vi "REC_magnet move program.vi"(4 "exp fit":cluster{"A":dbl, "B":dbl}={"A"=28.47, "B"=-1.501}, 5 "暂停磁铁引用":refnum<vi>, 6 "单次反馈":bool, 7 "反馈引用":refnum<vi>, 8 "预估时间引用":refnum<vi>, 9 "mag ctl":T1 {"磁铁运动参数"."FR每步时间(s)" min=0.5; "磁铁运动参数"."加载率(pN/s)" min=0.01}, 10 "停止测量引用":refnum<vi>, 11 "磁铁位置引用":refnum<vi>) -> (3 "完成测量":bool)   [LabVIEW 2017]
doc: "本VI是测量时控制磁铁运动的核心VI。\n不同的实验测量模式主要的区别就在于磁铁的运动过程不一样，因而在不同的测量模式下磁铁的运动模式也不同。\n必要的输入有：磁铁控制参数，临时终止测量，汇报磁铁位置。\n参数输入后首先会确定测量模式，然后敲定其他参数。\n目前完成的模式只有force clamp。\nFC的状态机逻辑如下：\n开始测量后，首先驰豫（可以设定驰豫位置），然后按位置数组和停留时间，顺序地走一遍，之后判断是否做往返，不做往返的话直接跳到完成检查阶段。如果做往返，跳转到返回运动，将数组反转后同样地走一遍，然后跳到完成检查阶段。完成检查阶段主要是判断是否测量了足够的周期，比如需要测两轮往返，那么在完成检查阶段就不会终止任务，而是跳转回到驰豫分支，开始一轮新的控制周期，直到完成了足够多的周期时，终止磁铁运动。"
uses:
  device control/magnet control.ctl
  device control/device index.ctl
  parameter set for record.ctl
  control/record mode.ctl
panel:
  # "force ramp"
  # "force ramp"
  # "通用"
  # "force ramp"
  # "force clamp"
  # "磁铁旋转"
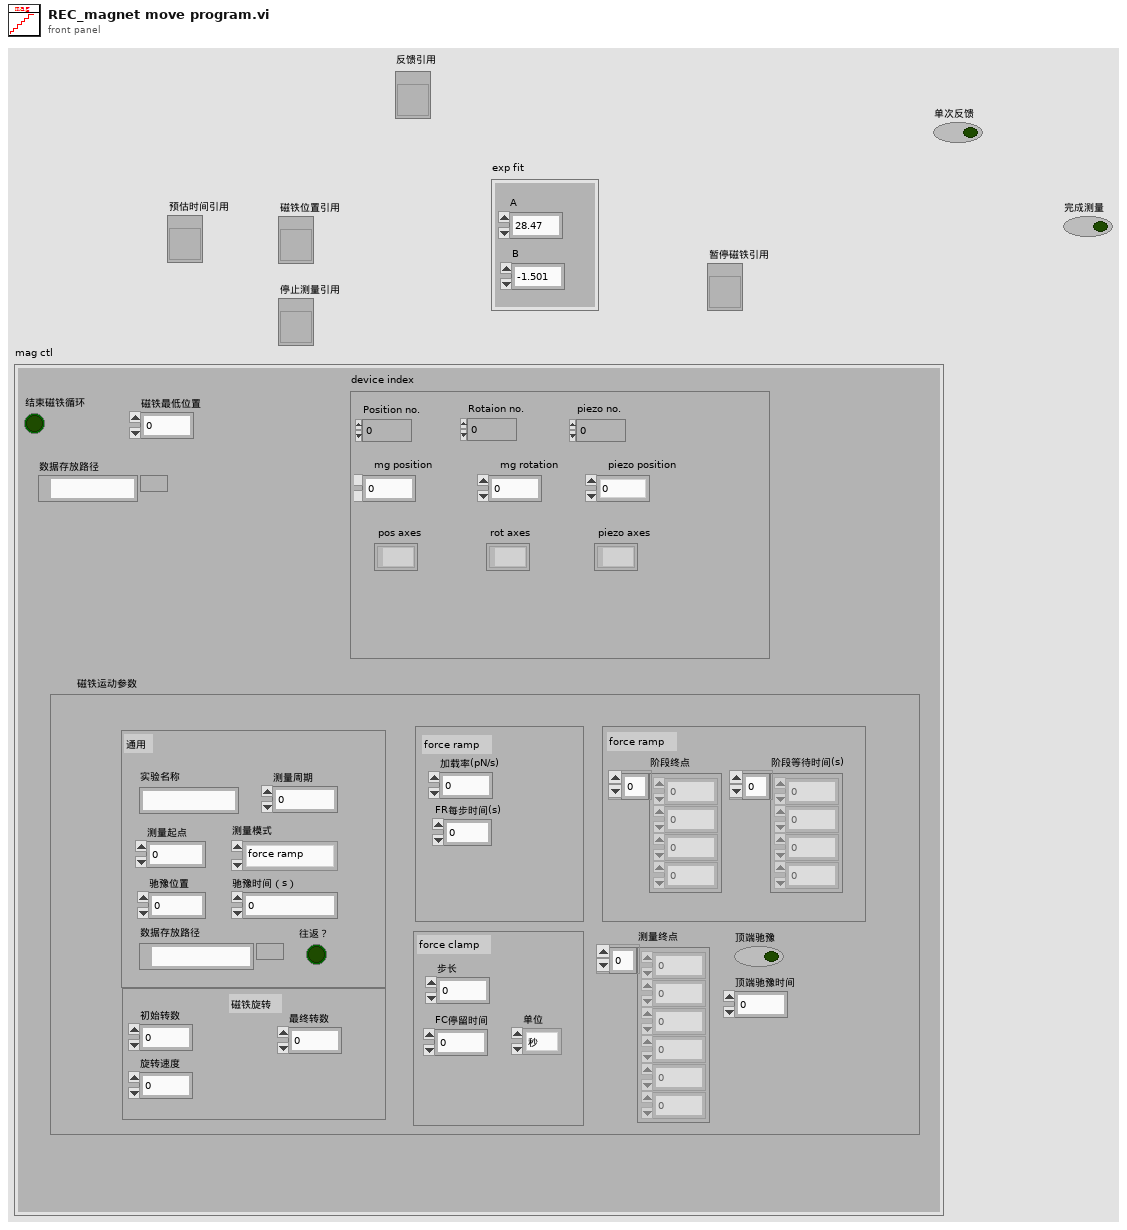
[diagram p1: front panel]
types:
  T1 = typedef "magnet control.ctl" = cluster{"device index":T2, "结束磁铁循环":bool, "磁铁最低位置":dbl, "数据存放路径":path, "磁铁运动参数":T3}
  T2 = typedef "device index.ctl" = cluster{"Position no.":i32, "Rotaion no.":i32, "piezo no.":i32, "mg position":dbl, "mg rotation":dbl, "piezo position":dbl, "pos axes":string[], "rot axes":string[], "piezo axes":string[]}
  T3 = typedef "parameter set for record.ctl" = cluster{"测量模式":T4, "测量起点":dbl, "数据存放路径":path, "加载率(pN/s)":dbl, "初始转数":dbl, "最终转数":dbl, "旋转速度":dbl, "步长":dbl, "FC停留时间":dbl, "实验名称":string, "往返？":bool, "驰豫时间（s）":dbl, "单位":enum16{"秒", "毫秒", "分"}, "测量周期":i32, "驰豫位置":dbl, "FR每步时间(s)":dbl, "测量终点":dbl[], "阶段终点":dbl[], "阶段等待时间(s)":dbl[], "顶端驰豫时间":u32, "顶端驰豫":bool}
  T4 = typedef "record mode.ctl" = enum16{"force ramp", "force clamp", "user-defined", "force-mixed"}
  T5 = typedef "磁铁进程控制变量.ctl" = enum16{"驰豫", "顺序运动", "返回运动", "完成检查"}
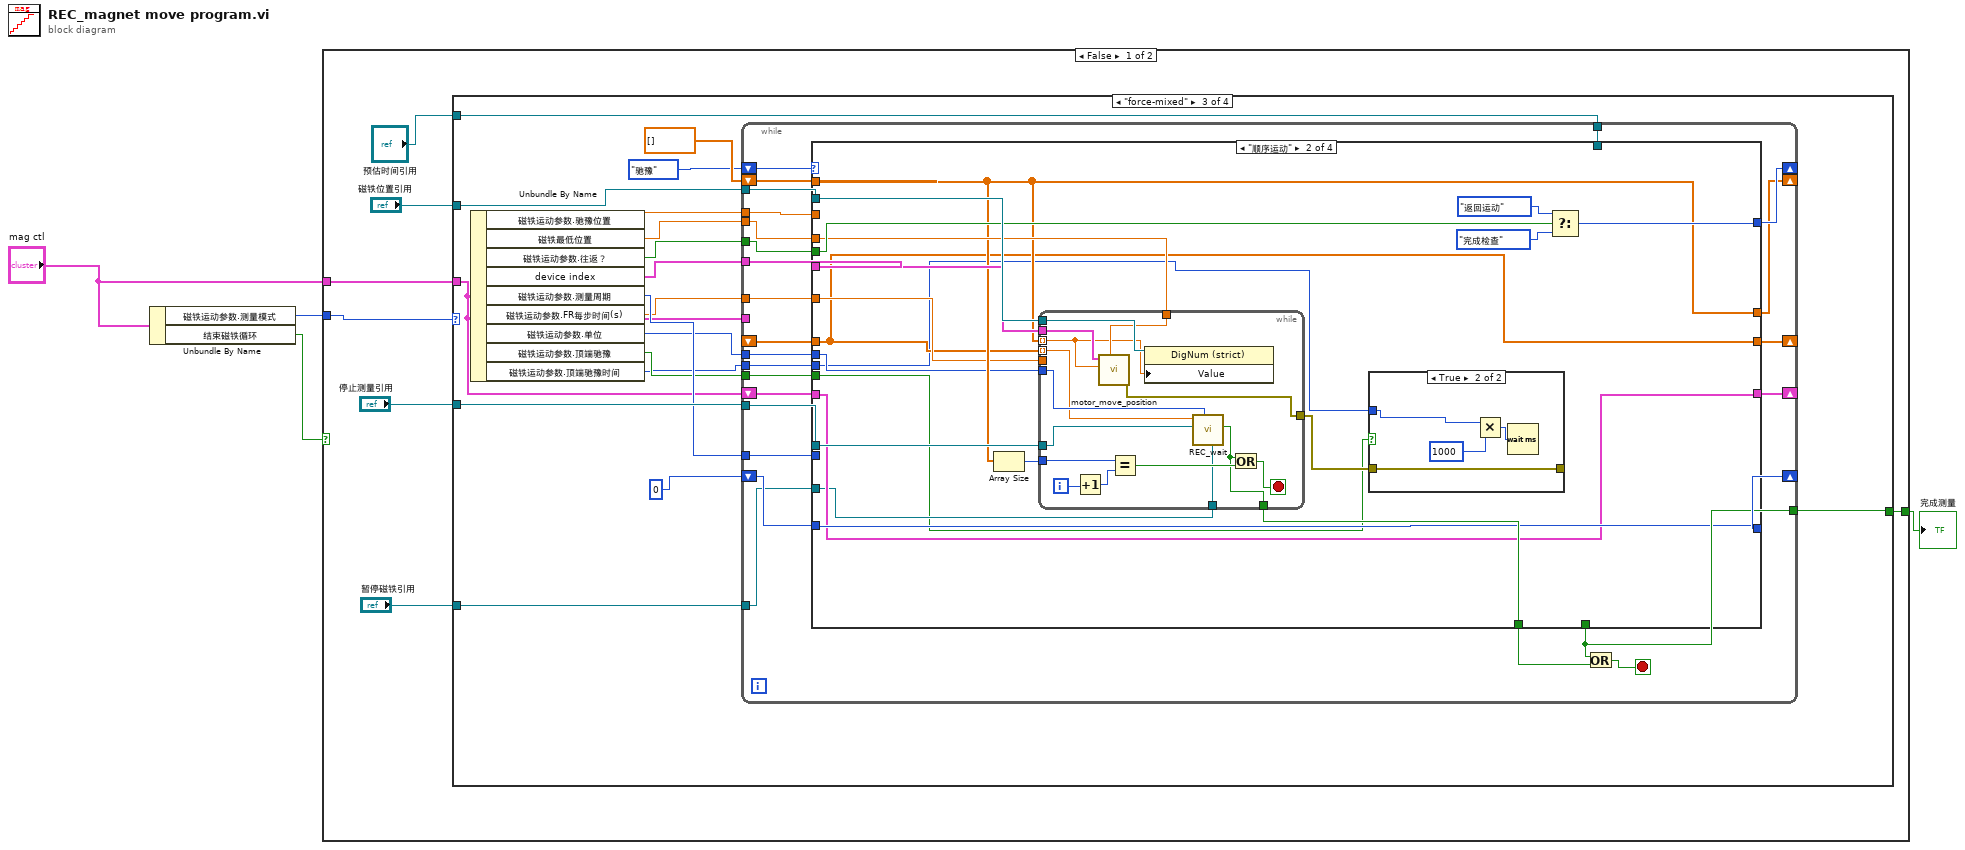
[diagram p0: block diagram]
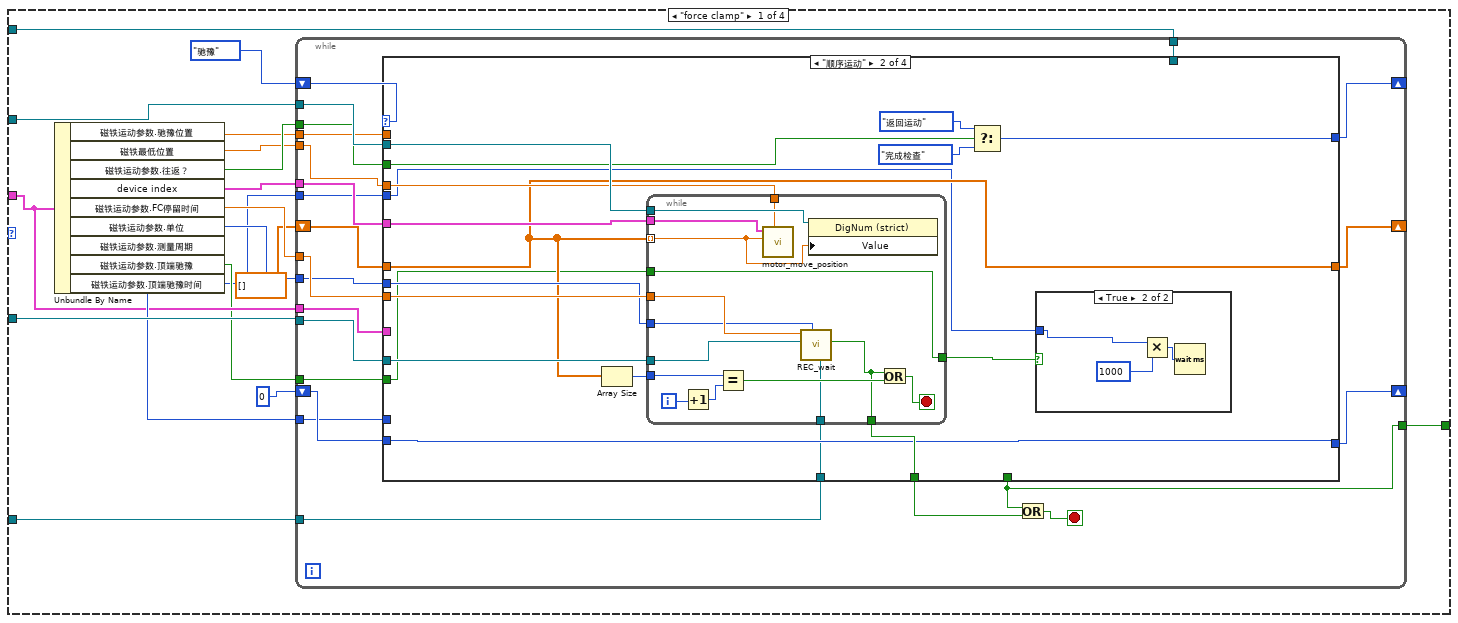
[diagram p2: hidden frame]
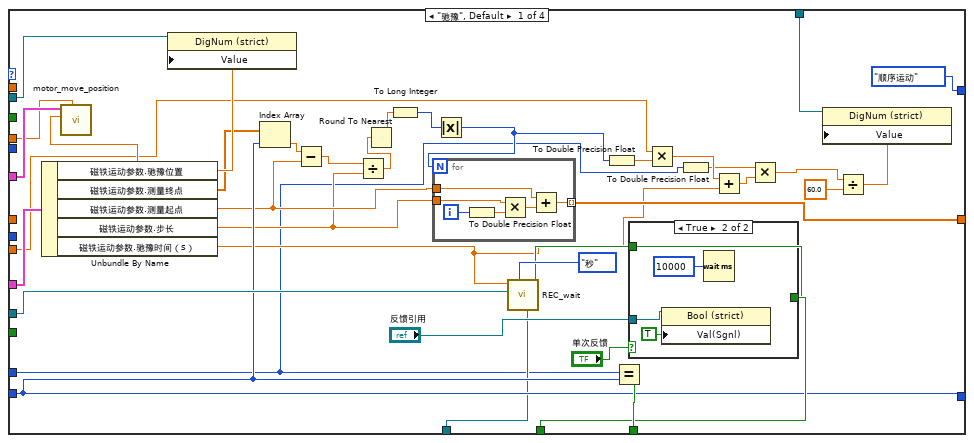
[diagram p3: hidden frame]
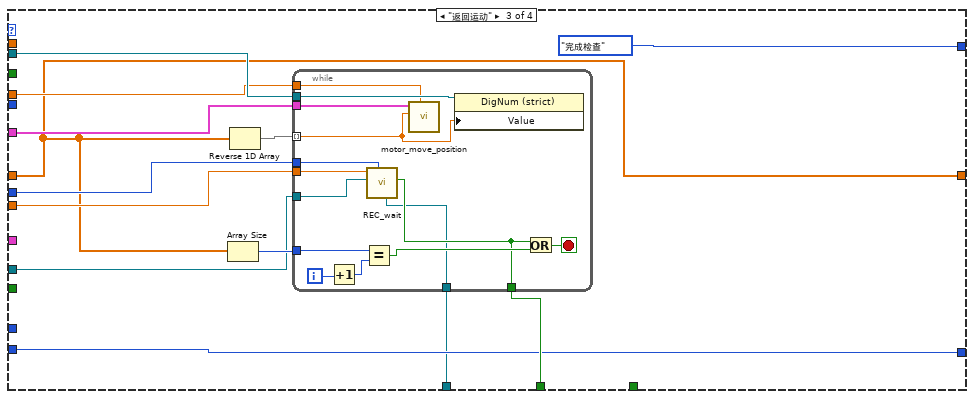
[diagram p6: hidden frame]
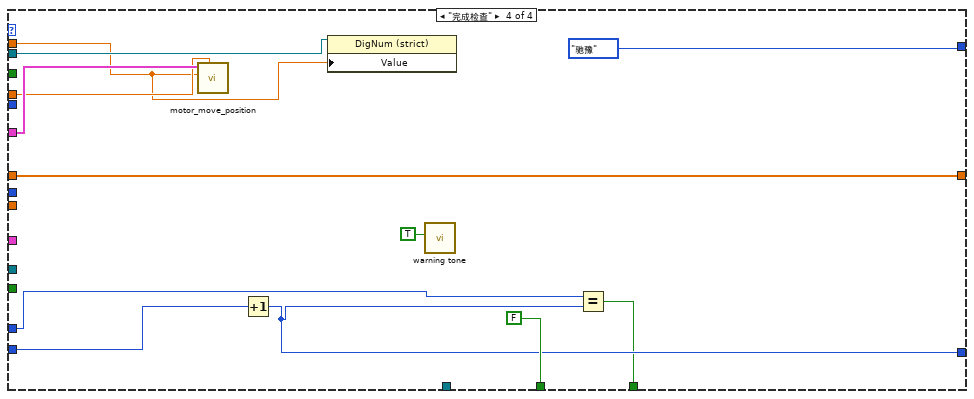
[diagram p7: hidden frame]
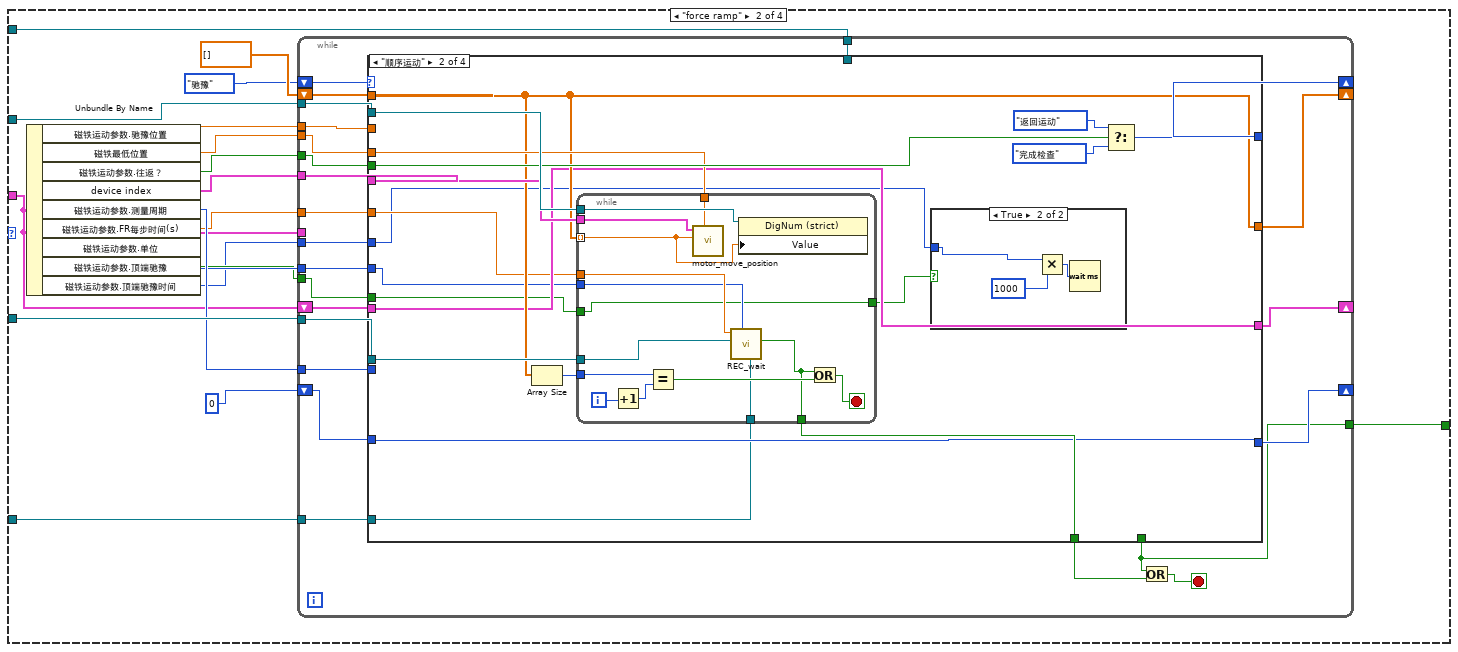
[diagram p8: hidden frame]
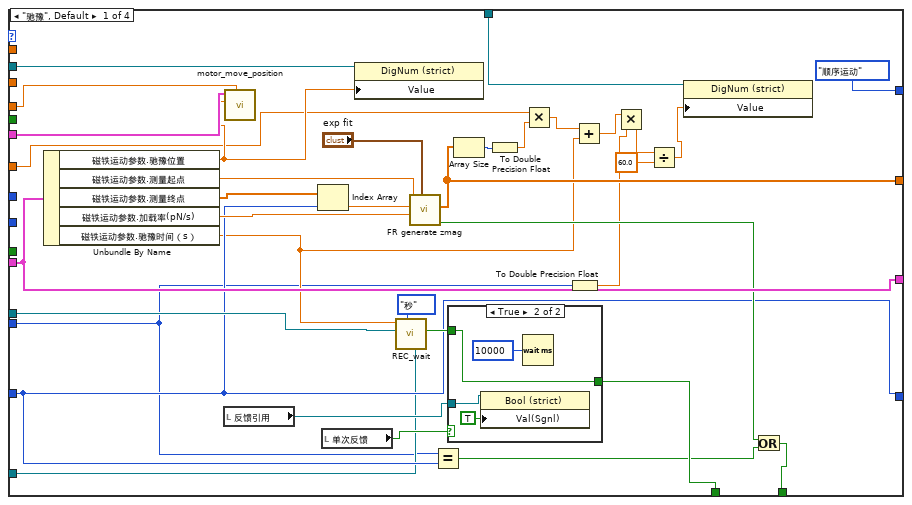
[diagram p9: hidden frame]
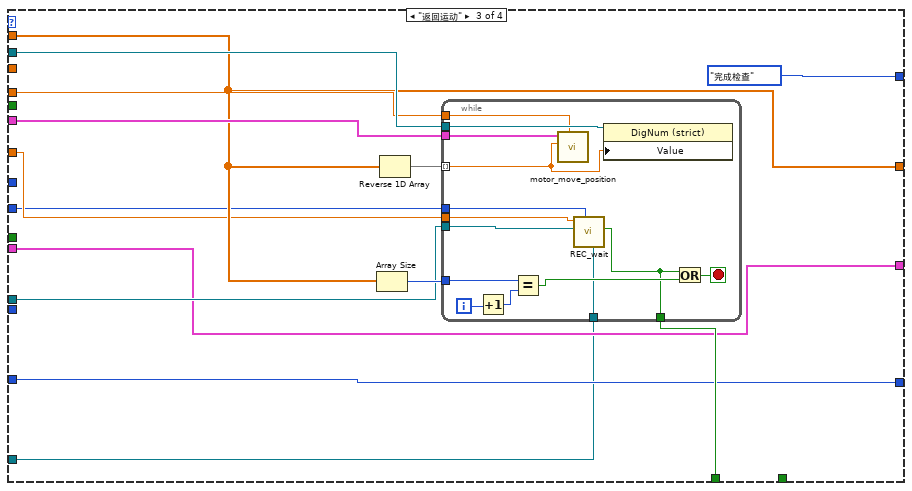
[diagram p12: hidden frame]
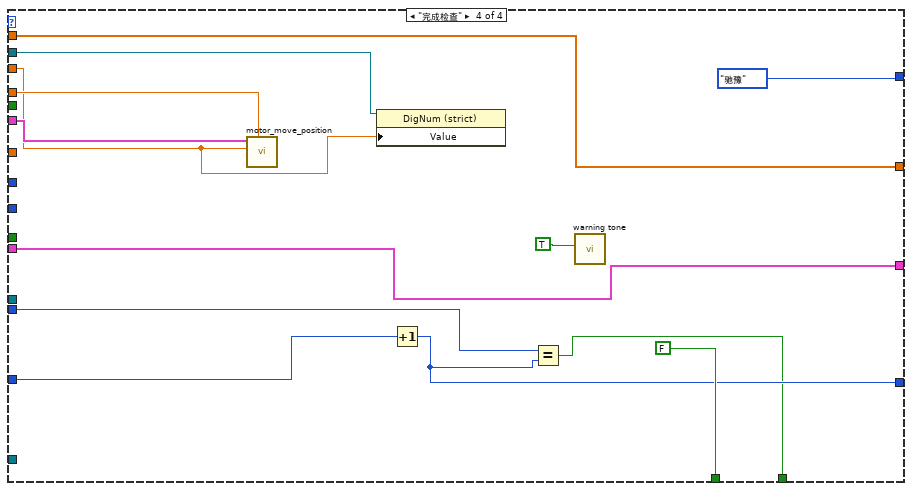
[diagram p13: hidden frame]
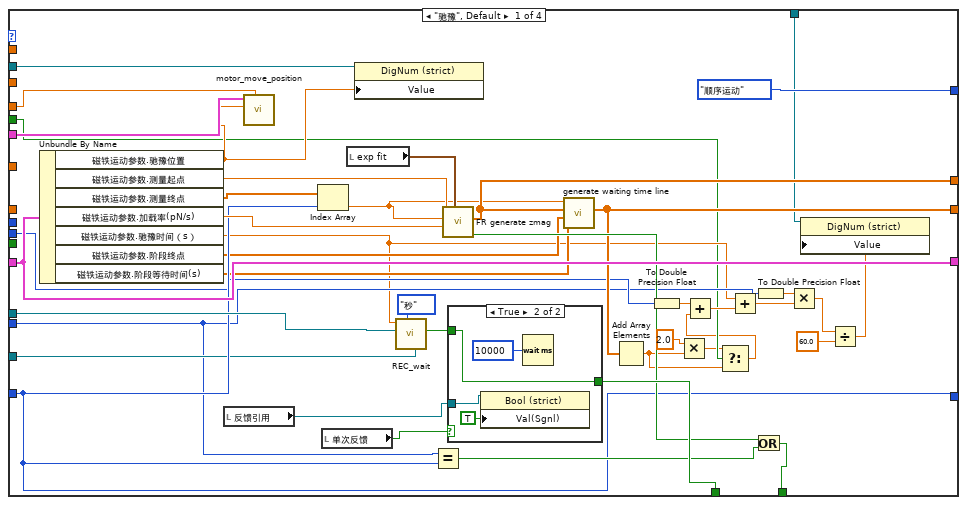
[diagram p14: hidden frame]
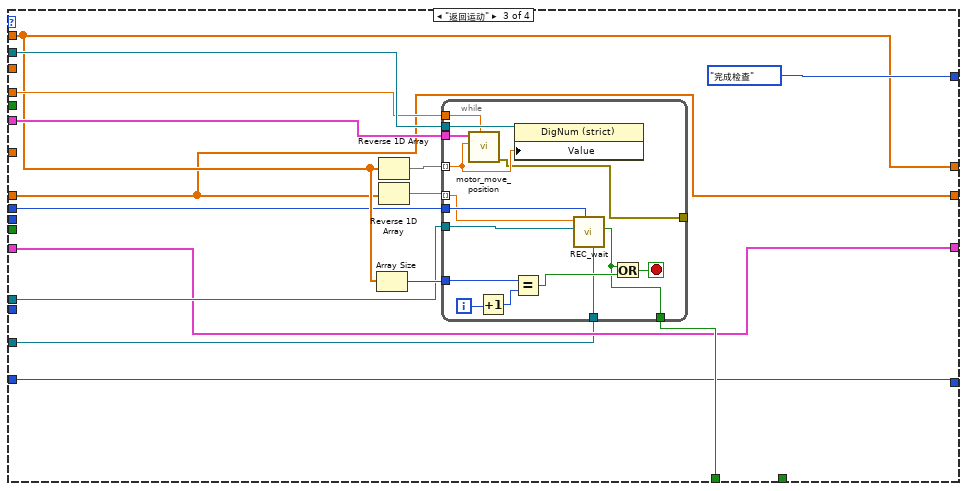
[diagram p17: hidden frame]
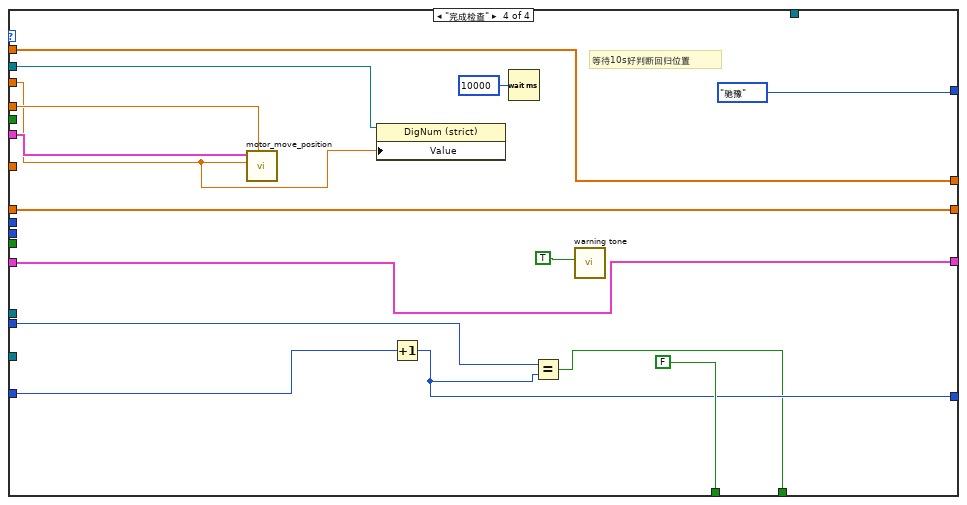
[diagram p18: hidden frame]
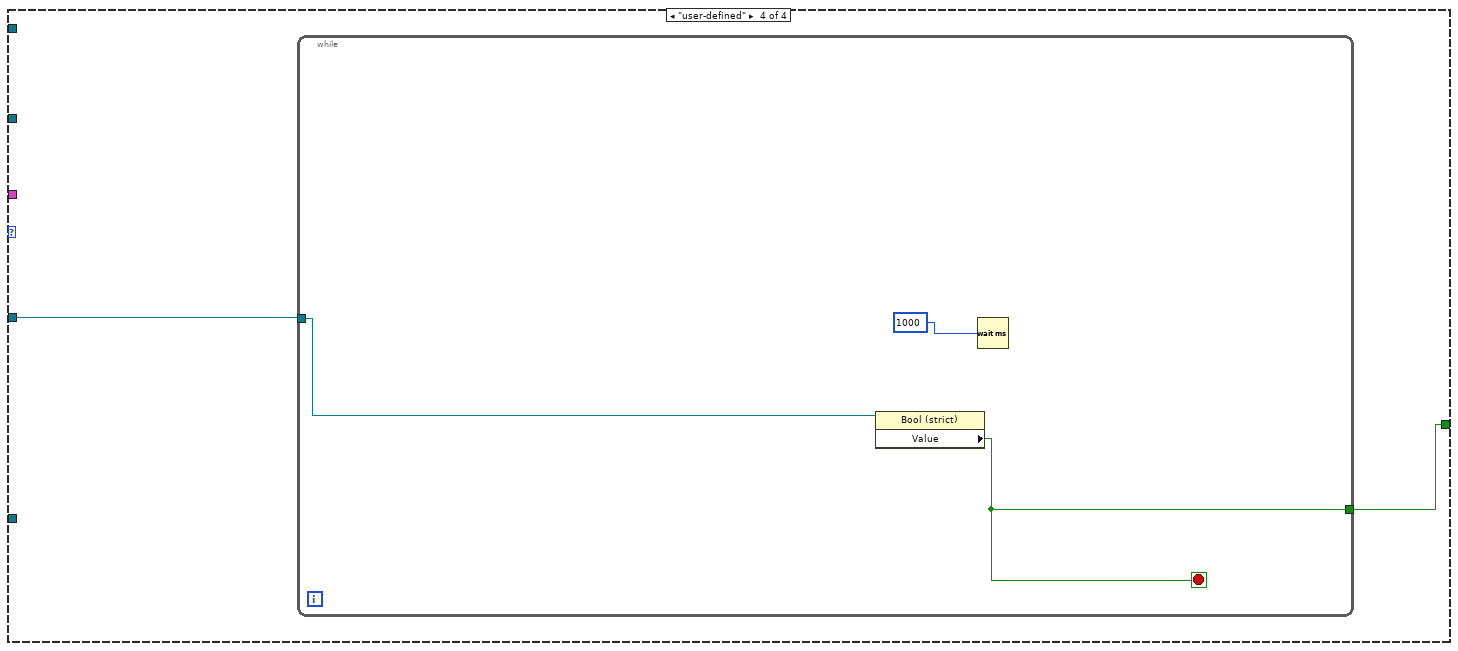
[diagram p19: hidden frame]
diagram:
  n1 = Unbundle By Name("mag ctl") -> ("磁铁运动参数.测量模式"=w4:T4, "结束磁铁循环"=w2:bool)
  n2 = case shown="False" w2 {
    selector: w2 -> [_ w516]
    tunnel: w4 -> [w11 _]
    tunnel: [w8 w516] -> w3
    tunnel: "mag ctl" -> [w7 _]
    frame False {
      n3 = case shown="\"force-mixed\"" w11 {
        tunnel: "磁铁位置引用" -> [w29 w189 w349 _]
        tunnel: "停止测量引用" -> [w28 w188 w348 w512]
        tunnel: w7 -> [w16 w183 w343 _]
        tunnel: [w21 w180 w340 w511] -> w8
        tunnel: "暂停磁铁引用" -> [w15 w178 w338 _]
        tunnel: "预估时间引用" -> [w14 w177 w335 _]
        frame "force clamp" {
          n4 = Unbundle By Name(w16) -> ("磁铁运动参数.驰豫位置"=w17:dbl, "磁铁最低位置"=w22:dbl, "磁铁运动参数.往返？"=w24:bool, "device index"=w26:T2, "磁铁运动参数.FC停留时间"=w25:dbl, "磁铁运动参数.单位"=w20:enum16{"秒", "毫秒", "分"}, "磁铁运动参数.测量周期"=w18:i32, "磁铁运动参数.顶端驰豫"=w13:bool, "磁铁运动参数.顶端驰豫时间"=w12:u32)
          n5 = while {
            tunnel: w29 -> [w52]
            tunnel: w28 -> [w51]
            shift-right: [w48] -> _
            shift-left: 磁铁进程控制变量."驰豫" -> [w49]
            tunnel: w26 -> [w47]
            tunnel: w25 -> [w46]
            tunnel: w24 -> [w45]
            shift-right: [w43] -> _
            shift-left: 0 -> [w44]
            tunnel: w22 -> [w42]
            tunnel: [w41] -> w21
            tunnel: w20 -> [w40]
            shift-right: [w39] -> _
            shift-left: dbl[] [] -> [w38]
            tunnel: w18 -> [w36]
            tunnel: w17 -> [w35]
            tunnel: w16 -> [w34]
            tunnel: w15 -> [w33]
            tunnel: w14 -> [w32]
            tunnel: w13 -> [w31]
            tunnel: w12 -> [w30]
            stop <- w50 stop-if-true
            n6 = case shown="\"顺序运动\"" w49 {
              tunnel: w52 -> [w84 w116 w142 w165]
              tunnel: w51 -> [w86 w115 w143 _]
              tunnel: [磁铁进程控制变量."顺序运动" w112 磁铁进程控制变量."完成检查" 磁铁进程控制变量."驰豫"] -> w48
              tunnel: [w81 w111 w146 FALSE ("Value")] -> w37
              tunnel: w47 -> [w85 w110 w144 w166]
              tunnel: w46 -> [w63 w109 w145 _]
              tunnel: w45 -> [_ w108 _ _]
              tunnel: w44 -> [w74 w107 w140 w172]
              tunnel: [w74 w107 w140 w169] -> w43
              tunnel: w42 -> [w83 w106 w139 w164]
              tunnel: [w82 _ _ w167] -> w41
              tunnel: w40 -> [_ w105 w138 _]
              tunnel: w34 -> [w68 _ _ _]
              tunnel: [w77 w104 w137 w171] -> w39
              tunnel: w38 -> [_ w104 w137 w171]
              tunnel: w36 -> [w58 _ _ w168]
              tunnel: w35 -> [_ _ _ w163]
              tunnel: w33 -> [w65 w103 w136 _]
              tunnel: w32 -> [w56 _ _ _]
              tunnel: w31 -> [_ w101 _ _]
              tunnel: w30 -> [_ w102 _ _]
              frame "驰豫", Default {
                n7 = Unbundle By Name(w68) -> ("磁铁运动参数.驰豫位置"=w78:dbl, "磁铁运动参数.测量终点"=w75:dbl[], "磁铁运动参数.测量起点"=w72:dbl, "磁铁运动参数.步长"=w71:dbl, "磁铁运动参数.驰豫时间（s）"=w64:dbl)
                n8 = call "motor_move_position.vi"("磁铁最低位置"=w83, "target position"=w78, "device index"=w85) -> ()  [unwired: 6 in, 3 out]
                n9 = property class="DigNum (strict)"(reference=w84, "Value"=w78) -> ()  [unwired: 1 in, 2 out]
                n10 = Index Array(array=w75, index=w74) -> (element=w73:dbl)
                n11 = Subtract(x=w73, y=w72) -> (x-y=w66:dbl)
                n12 = Divide(x=w66, y=w71) -> (x/y=w70:dbl)
                n13 = Round To Nearest(number=w70) -> (nearest integer value=w69:dbl)
                n14 = To Long Integer(number=w69) -> (32bit integer=w67:i32)
                n15 = Absolute Value(x=w67) -> (abs(x)=w62:i32)
                n16 = for {
                  N: w62 -> [_]
                  tunnel: w72 -> [w94]
                  tunnel: [w90] -> w77 mode=indexing
                  tunnel: w71 -> [w89]
                  i -> [w93]
                  n17 = To Double Precision Float(number=w93) -> (double precision float=w92:dbl)
                  n18 = Multiply(x=w89, y=w92) -> (x*y=w91:dbl)
                  n19 = Add(x=w94, y=w91) -> (x+y=w90:dbl)
                }
                n20 = call "REC_wait.vi"("暂停磁铁引用"=w65, "时间单位"=enum16{"秒", "毫秒", "分"}."秒", "停止测量引用"=w86, "停留时间"=w64) -> ("停止？"=w80:bool)  [unwired: 7 in]
                n21 = To Double Precision Float(number=w62) -> (double precision float=w61:dbl)
                n22 = Equal?(x=w58, y=w74) -> (x = y?=w82:bool)
                n23 = case shown="True" "单次反馈" {
                  selector: "单次反馈" -> [w95 _]
                  tunnel: [w95 w97] -> w81
                  tunnel: w80 -> [_ w97]
                  tunnel: "反馈引用" -> [_ w96]
                  frame False {
                  }
                  frame True {
                    n24 = property class="Bool (strict)"(reference=w96, "Val(Sgnl)"=TRUE ("值(信号)")) -> ()  [unwired: 1 in, 2 out]
                    n25 = Wait (ms)(milliseconds to wait=u32 10000 ("等待时间（毫秒）")) -> ()  [unwired: 1 out]
                  }
                }
                n26 = Multiply(x=w63, y=w61) -> (x*y=w60:dbl)
                n27 = To Double Precision Float(number=w58) -> (double precision float=w57:dbl)
                n28 = Add(x=w60, y=w64) -> (x+y=w59:dbl)
                n29 = Multiply(x=w57, y=w59) -> (x*y=w54:dbl)
                n30 = Divide(x=w54, y=60.0) -> (x/y=w53:dbl)
                n31 = property class="DigNum (strict)"(reference=w56, "Value"=w53) -> ()  [unwired: 1 in, 2 out]
              }
              frame "顺序运动" {
                n32 = Array Size(array=w104) -> (size(s)=w117:i32)
                n33 = while {
                  tunnel: w117 -> [w135]
                  tunnel: w116 -> [w130]
                  tunnel: w115 -> [w127]
                  tunnel: [w126] -> w111
                  tunnel: w110 -> [w129]
                  tunnel: w109 -> [w128]
                  tunnel: w106 -> [w125]
                  tunnel: w105 -> [w124]
                  tunnel: w104 -> [w123] mode=indexing
                  tunnel: w103 -> [w122]
                  tunnel: [w121] -> w100
                  tunnel: w101 -> [w121]
                  i -> [w134]
                  stop <- w132 stop-if-true
                  n34 = Increment(x=w134) -> (x+1=w133:i32)
                  n35 = Equal?(x=w135, y=w133) -> (x = y?=w131:bool)
                  n36 = call "motor_move_position.vi"("磁铁最低位置"=w125, "target position"=w123, "device index"=w129) -> ()  [unwired: 6 in, 3 out]
                  n37 = call "REC_wait.vi"("暂停磁铁引用"=w122, "时间单位"=w124, "停止测量引用"=w127, "停留时间"=w128) -> ("停止？"=w126:bool)  [unwired: 7 in]
                  n38 = property class="DigNum (strict)"(reference=w130, "Value"=w123) -> ()  [unwired: 1 in, 2 out]
                  n39 = Or(x=w126, y=w131) -> (x .or. y?=w132:bool)
                }
                n40 = Select(t=磁铁进程控制变量."返回运动", s=w108, f=磁铁进程控制变量."完成检查") -> (s? t:f=w112:T5)
                n41 = case shown="True" w100 {
                  tunnel: w102 -> [_ w118]
                  frame False {
                  }
                  frame True {
                    n42 = Multiply(x=w118, y=u32 1000) -> (x*y=w119:u32)
                    n43 = Wait (ms)(milliseconds to wait=w119) -> ()  [unwired: 1 out]
                  }
                }
              }
              frame "返回运动" {
                n44 = Array Size(array=w137) -> (size(s)=w147:i32)
                n45 = Reverse 1D Array(array=w137) -> (reversed array=w148:dbl[])
                n46 = while {
                  tunnel: [w153] -> w146
                  tunnel: w148 -> [w151] mode=indexing
                  tunnel: w147 -> [w158]
                  tunnel: w145 -> [w157]
                  tunnel: w144 -> [w156]
                  tunnel: w143 -> [w154]
                  tunnel: w142 -> [w155]
                  tunnel: w139 -> [w152]
                  tunnel: w138 -> [w150]
                  tunnel: w136 -> [w149]
                  i -> [w162]
                  stop <- w160 stop-if-true
                  n47 = Increment(x=w162) -> (x+1=w161:i32)
                  n48 = Equal?(x=w158, y=w161) -> (x = y?=w159:bool)
                  n49 = call "REC_wait.vi"("暂停磁铁引用"=w149, "时间单位"=w150, "停止测量引用"=w154, "停留时间"=w157) -> ("停止？"=w153:bool)  [unwired: 7 in]
                  n50 = call "motor_move_position.vi"("磁铁最低位置"=w152, "target position"=w151, "device index"=w156) -> ()  [unwired: 6 in, 3 out]
                  n51 = property class="DigNum (strict)"(reference=w155, "Value"=w151) -> ()  [unwired: 1 in, 2 out]
                  n52 = Or(x=w153, y=w159) -> (x .or. y?=w160:bool)
                }
              }
              frame "完成检查" {
                n53 = call "motor_move_position.vi"("磁铁最低位置"=w164, "target position"=w163, "device index"=w166) -> ()  [unwired: 6 in, 3 out]
                n54 = Increment(x=w172) -> (x+1=w169:i32)
                n55 = property class="DigNum (strict)"(reference=w165, "Value"=w163) -> ()  [unwired: 1 in, 2 out]
                n56 = call "warning tone.vi"("Ring?"=TRUE) -> ()  [unwired: 11 in]
                n57 = Equal?(x=w168, y=w169) -> (x = y?=w167:bool)
              }
            }
            n58 = Or(x=w41, y=w37) -> (x .or. y?=w50:bool)
          }
        }
        frame "force ramp" {
          n59 = Unbundle By Name(w183) -> ("磁铁运动参数.驰豫位置"=w179:dbl, "磁铁最低位置"=w191:dbl, "磁铁运动参数.往返？"=w190:bool, "device index"=w192:T2, "磁铁运动参数.测量周期"=w185:i32, "磁铁运动参数.FR每步时间(s)"=w182:dbl, "磁铁运动参数.单位"=w181:enum16{"秒", "毫秒", "分"}, "磁铁运动参数.顶端驰豫"=w176:bool, "磁铁运动参数.顶端驰豫时间"=w175:u32)
          n60 = while {
            tunnel: w189 -> [w216]
            tunnel: w188 -> [w215]
            shift-right: [w212] -> _
            shift-left: 磁铁进程控制变量."驰豫" -> [w213]
            tunnel: w192 -> [w210]
            tunnel: w190 -> [w209]
            shift-right: [w207] -> _
            shift-left: 0 -> [w208]
            tunnel: [w206] -> w180
            shift-right: [w205] -> _
            shift-left: w183 -> [w200]
            shift-right: [w204] -> _
            shift-left: dbl[] [] -> [w203]
            tunnel: w191 -> [w202]
            tunnel: w185 -> [w201]
            tunnel: w183 -> [_]
            tunnel: w182 -> [w199]
            tunnel: w181 -> [w198]
            tunnel: w179 -> [w197]
            tunnel: w178 -> [w196]
            tunnel: w177 -> [w195]
            tunnel: w176 -> [w194]
            tunnel: w175 -> [w193]
            stop <- w214 stop-if-true
            n61 = case shown="\"顺序运动\"" w213 {
              tunnel: w216 -> [w247 w274 w302 w322]
              tunnel: w215 -> [w249 w273 w303 _]
              tunnel: [磁铁进程控制变量."顺序运动" w270 磁铁进程控制变量."完成检查" 磁铁进程控制变量."驰豫"] -> w212
              tunnel: [w238 w269 w305 FALSE ("Value")] -> w211
              tunnel: w210 -> [w248 w268 w304 w325]
              tunnel: w209 -> [_ w267 _ _]
              tunnel: w208 -> [w231 w266 w300 w332]
              tunnel: [w231 w266 w300 w328] -> w207
              tunnel: w202 -> [w246 w265 w299 w324]
              tunnel: [w235 _ _ w326] -> w206
              tunnel: w200 -> [w241 w263 w298 w331]
              tunnel: [w241 w263 w298 w331] -> w205
              tunnel: [w229 w264 w297 w330] -> w204
              tunnel: w203 -> [_ w264 w297 w330]
              tunnel: w201 -> [w222 _ _ w327]
              tunnel: w199 -> [w228 w262 w296 _]
              tunnel: w198 -> [_ w261 w295 _]
              tunnel: w197 -> [_ _ _ w323]
              tunnel: w196 -> [w230 w260 w294 _]
              tunnel: w195 -> [w217 _ _ _]
              tunnel: w194 -> [_ w259 _ _]
              tunnel: w193 -> [_ w257 _ _]
              frame "驰豫", Default {
                n62 = Unbundle By Name(w241) -> ("磁铁运动参数.驰豫位置"=w242:dbl, "磁铁运动参数.测量起点"=w240:dbl, "磁铁运动参数.测量终点"=w233:dbl[], "磁铁运动参数.加载率(pN/s)"=w239:dbl, "磁铁运动参数.驰豫时间（s）"=w224:dbl)
                n63 = local read "反馈引用"() -> (w244:refnum<vi>)
                n64 = call "motor_move_position.vi"("磁铁最低位置"=w246, "target position"=w242, "device index"=w248) -> ()  [unwired: 6 in, 3 out]
                n65 = Index Array(array=w233, index=w231) -> (element=w232:dbl)
                n66 = local read "单次反馈"() -> (w243:bool)
                n67 = property class="DigNum (strict)"(reference=w247, "Value"=w242) -> ()  [unwired: 1 in, 2 out]
                n68 = call "REC_wait.vi"("暂停磁铁引用"=w230, "时间单位"=enum16{"秒", "毫秒", "分"}."秒", "停止测量引用"=w249, "停留时间"=w224) -> ("停止？"=w245:bool)  [unwired: 7 in]
                n69 = call "FR generate zmag.vi"("exp fit"="exp fit", "每步加载率"=w239, "终点"=w232, "起点"=w240) -> ("Wrong"=w236:bool, "FR zmag"=w229:dbl[])  [unwired: 6 in]
                n70 = Equal?(x=w222, y=w231) -> (x = y?=w237:bool)
                n71 = case shown="True" w243 {
                  selector: w243 -> [w252 _]
                  tunnel: [w252 w254] -> w238
                  tunnel: w245 -> [_ w254]
                  tunnel: w244 -> [_ w253]
                  frame False {
                  }
                  frame True {
                    n72 = property class="Bool (strict)"(reference=w253, "Val(Sgnl)"=TRUE ("值(信号)")) -> ()  [unwired: 1 in, 2 out]
                    n73 = Wait (ms)(milliseconds to wait=u32 10000 ("等待时间（毫秒）")) -> ()  [unwired: 1 out]
                  }
                }
                n74 = Array Size(array=w229) -> (size(s)=w227:i32)
                n75 = To Double Precision Float(number=w227) -> (double precision float=w226:dbl)
                n76 = Multiply(x=w228, y=w226) -> (x*y=w225:dbl)
                n77 = To Double Precision Float(number=w222) -> (double precision float=w221:dbl)
                n78 = Add(x=w225, y=w224) -> (x+y=w223:dbl)
                n79 = Multiply(x=w223, y=w221) -> (x*y=w220:dbl)
                n80 = Divide(x=w220, y=60.0) -> (x/y=w218:dbl)
                n81 = property class="DigNum (strict)"(reference=w217, "Value"=w218) -> ()  [unwired: 1 in, 2 out]
                n82 = Or(x=w236, y=w237) -> (x .or. y?=w235:bool)
              }
              frame "顺序运动" {
                n83 = Array Size(array=w264) -> (size(s)=w275:i32)
                n84 = while {
                  tunnel: w275 -> [w293]
                  tunnel: w274 -> [w288]
                  tunnel: w273 -> [w286]
                  tunnel: [w285] -> w269
                  tunnel: w268 -> [w287]
                  tunnel: w265 -> [w284]
                  tunnel: w264 -> [w283] mode=indexing
                  tunnel: w262 -> [w282]
                  tunnel: w261 -> [w281]
                  tunnel: w260 -> [w280]
                  tunnel: w259 -> [w279]
                  tunnel: [w279] -> w258
                  i -> [w292]
                  stop <- w290 stop-if-true
                  n85 = Increment(x=w292) -> (x+1=w291:i32)
                  n86 = Equal?(x=w293, y=w291) -> (x = y?=w289:bool)
                  n87 = call "motor_move_position.vi"("磁铁最低位置"=w284, "target position"=w283, "device index"=w287) -> ()  [unwired: 6 in, 3 out]
                  n88 = call "REC_wait.vi"("暂停磁铁引用"=w280, "时间单位"=w281, "停止测量引用"=w286, "停留时间"=w282) -> ("停止？"=w285:bool)  [unwired: 7 in]
                  n89 = property class="DigNum (strict)"(reference=w288, "Value"=w283) -> ()  [unwired: 1 in, 2 out]
                  n90 = Or(x=w285, y=w289) -> (x .or. y?=w290:bool)
                }
                n91 = case shown="True" w258 {
                  tunnel: w257 -> [_ w276]
                  frame False {
                  }
                  frame True {
                    n92 = Multiply(x=w276, y=u32 1000) -> (x*y=w277:u32)
                    n93 = Wait (ms)(milliseconds to wait=w277) -> ()  [unwired: 1 out]
                  }
                }
                n94 = Select(t=磁铁进程控制变量."返回运动", s=w267, f=磁铁进程控制变量."完成检查") -> (s? t:f=w270:T5)
              }
              frame "返回运动" {
                n95 = Array Size(array=w297) -> (size(s)=w306:i32)
                n96 = Reverse 1D Array(array=w297) -> (reversed array=w307:dbl[])
                n97 = while {
                  tunnel: [w313] -> w305
                  tunnel: w307 -> [w311] mode=indexing
                  tunnel: w306 -> [w317]
                  tunnel: w304 -> [w316]
                  tunnel: w303 -> [w314]
                  tunnel: w302 -> [w315]
                  tunnel: w299 -> [w312]
                  tunnel: w296 -> [w310]
                  tunnel: w295 -> [w309]
                  tunnel: w294 -> [w308]
                  i -> [w321]
                  stop <- w319 stop-if-true
                  n98 = Increment(x=w321) -> (x+1=w320:i32)
                  n99 = Equal?(x=w317, y=w320) -> (x = y?=w318:bool)
                  n100 = call "motor_move_position.vi"("磁铁最低位置"=w312, "target position"=w311, "device index"=w316) -> ()  [unwired: 6 in, 3 out]
                  n101 = call "REC_wait.vi"("暂停磁铁引用"=w308, "时间单位"=w309, "停止测量引用"=w314, "停留时间"=w310) -> ("停止？"=w313:bool)  [unwired: 7 in]
                  n102 = property class="DigNum (strict)"(reference=w315, "Value"=w311) -> ()  [unwired: 1 in, 2 out]
                  n103 = Or(x=w313, y=w318) -> (x .or. y?=w319:bool)
                }
              }
              frame "完成检查" {
                n104 = call "motor_move_position.vi"("磁铁最低位置"=w324, "target position"=w323, "device index"=w325) -> ()  [unwired: 6 in, 3 out]
                n105 = property class="DigNum (strict)"(reference=w322, "Value"=w323) -> ()  [unwired: 1 in, 2 out]
                n106 = Increment(x=w332) -> (x+1=w328:i32)
                n107 = Equal?(x=w327, y=w328) -> (x = y?=w326:bool)
                n108 = call "warning tone.vi"("Ring?"=TRUE) -> ()  [unwired: 11 in]
              }
            }
            n109 = Or(x=w206, y=w211) -> (x .or. y?=w214:bool)
          }
        }
        frame "force-mixed" {
          n110 = Unbundle By Name(w343) -> ("磁铁运动参数.驰豫位置"=w339:dbl, "磁铁最低位置"=w351:dbl, "磁铁运动参数.往返？"=w350:bool, "device index"=w352:T2, "磁铁运动参数.测量周期"=w345:i32, "磁铁运动参数.FR每步时间(s)"=w342:dbl, "磁铁运动参数.单位"=w341:enum16{"秒", "毫秒", "分"}, "磁铁运动参数.顶端驰豫"=w337:bool, "磁铁运动参数.顶端驰豫时间"=w336:u32)
          n111 = while {
            tunnel: w349 -> [w378]
            tunnel: w348 -> [w377]
            shift-right: [w374] -> _
            shift-left: 磁铁进程控制变量."驰豫" -> [w375]
            tunnel: w352 -> [w372]
            tunnel: w350 -> [w371]
            shift-right: [w369] -> _
            shift-left: 0 -> [w370]
            tunnel: [w368] -> w340
            shift-right: [w367] -> _
            shift-left: w343 -> [w362]
            shift-right: [w366] -> _
            shift-left: dbl[] [] -> [w365]
            tunnel: w351 -> [w364]
            tunnel: w345 -> [w363]
            tunnel: w343 -> [_]
            tunnel: w342 -> [w361]
            tunnel: w341 -> [w360]
            tunnel: w339 -> [w359]
            shift-right: [w358] -> _
            shift-left: _ -> [w357]
            tunnel: w338 -> [w356]
            tunnel: w337 -> [w355]
            tunnel: w336 -> [w354]
            tunnel: w335 -> [w353]
            stop <- w376 stop-if-true
            n112 = case shown="\"顺序运动\"" w375 {
              tunnel: w378 -> [w416 w444 w475 w498]
              tunnel: w377 -> [w418 w443 w476 _]
              tunnel: [磁铁进程控制变量."顺序运动" w440 磁铁进程控制变量."完成检查" 磁铁进程控制变量."驰豫"] -> w374
              tunnel: [w407 w439 w478 FALSE ("Value")] -> w373
              tunnel: w372 -> [w417 w438 w477 w501]
              tunnel: w371 -> [w387 w437 _ _]
              tunnel: w370 -> [w402 w436 w473 w508]
              tunnel: [w402 w436 w473 w504] -> w369
              tunnel: w364 -> [w415 w435 w472 w500]
              tunnel: [w404 _ _ w502] -> w368
              tunnel: w362 -> [w410 w433 w471 w507]
              tunnel: [w410 w433 w471 w507] -> w367
              tunnel: [w400 w434 w470 w506] -> w366
              tunnel: w365 -> [_ w434 w470 w506]
              tunnel: w363 -> [w392 _ _ w503]
              tunnel: w361 -> [_ w432 _ _]
              tunnel: w360 -> [_ w431 w469 _]
              tunnel: w359 -> [_ _ _ w499]
              tunnel: [w395 w430 w466 w497] -> w358
              tunnel: w357 -> [_ w430 w466 w497]
              tunnel: w356 -> [w396 w429 w468 _]
              tunnel: w355 -> [_ w427 _ _]
              tunnel: w354 -> [w394 w426 _ _]
              tunnel: w353 -> [w379 _ _ _]
              frame "驰豫", Default {
                n113 = Unbundle By Name(w410) -> ("磁铁运动参数.驰豫位置"=w411:dbl, "磁铁运动参数.测量起点"=w409:dbl, "磁铁运动参数.测量终点"=w403:dbl[], "磁铁运动参数.加载率(pN/s)"=w408:dbl, "磁铁运动参数.驰豫时间（s）"=w390:dbl, "磁铁运动参数.阶段终点"=w399:dbl[], "磁铁运动参数.阶段等待时间(s)"=w398:dbl[])
                n114 = local read "反馈引用"() -> (w413:refnum<vi>)
                n115 = call "motor_move_position.vi"("磁铁最低位置"=w415, "target position"=w411, "device index"=w417) -> ()  [unwired: 6 in, 3 out]
                n116 = Index Array(array=w403, index=w402) -> (element=w397:dbl)
                n117 = local read "单次反馈"() -> (w412:bool)
                n118 = local read "exp fit"() -> (w401:cluster{"A":dbl, "B":dbl})
                n119 = property class="DigNum (strict)"(reference=w416, "Value"=w411) -> ()  [unwired: 1 in, 2 out]
                n120 = call "REC_wait.vi"("暂停磁铁引用"=w396, "时间单位"=enum16{"秒", "毫秒", "分"}."秒", "停止测量引用"=w418, "停留时间"=w390) -> ("停止？"=w414:bool)  [unwired: 7 in]
                n121 = Equal?(x=w392, y=w402) -> (x = y?=w406:bool)
                n122 = call "FR generate zmag.vi"("exp fit"=w401, "每步加载率"=w408, "终点"=w397, "起点"=w409) -> ("Wrong"=w405:bool, "FR zmag"=w400:dbl[])  [unwired: 6 in]
                n123 = case shown="True" w412 {
                  selector: w412 -> [w421 _]
                  tunnel: [w421 w423] -> w407
                  tunnel: w414 -> [_ w423]
                  tunnel: w413 -> [_ w422]
                  frame False {
                  }
                  frame True {
                    n124 = property class="Bool (strict)"(reference=w422, "Val(Sgnl)"=TRUE ("值(信号)")) -> ()  [unwired: 1 in, 2 out]
                    n125 = Wait (ms)(milliseconds to wait=u32 10000 ("等待时间（毫秒）")) -> ()  [unwired: 1 out]
                  }
                }
                n126 = call "generate waiting time line.vi"("每步等待时间(s)"=w398, "阶段终点"=w399, "FR zmag"=w400, "真 终点"=w397) -> ("FR time line"=w395:dbl[])  [unwired: 7 in]
                n127 = Add Array Elements(numeric array=w395) -> (sum=w384:dbl)
                n128 = To Double Precision Float(number=w394) -> (double precision float=w393:dbl)
                n129 = Multiply(x=2.0, y=w384) -> (x*y=w386:dbl)
                n130 = Select(t=w386, s=w387, f=w384) -> (s? t:f=w383:dbl)
                n131 = Add(x=w393, y=w383) -> (x+y=w389:dbl)
                n132 = Add(x=w390, y=w389) -> (x+y=w388:dbl)
                n133 = Or(x=w405, y=w406) -> (x .or. y?=w404:bool)
                n134 = To Double Precision Float(number=w392) -> (double precision float=w391:dbl)
                n135 = Multiply(x=w391, y=w388) -> (x*y=w382:dbl)
                n136 = Divide(x=w382, y=60.0) -> (x/y=w380:dbl)
                n137 = property class="DigNum (strict)"(reference=w379, "Value"=w380) -> ()  [unwired: 1 in, 2 out]
              }
              frame "顺序运动" {
                n138 = Array Size(array=w434) -> (size(s)=w445:i32)
                n139 = while {
                  tunnel: w445 -> [w465]
                  tunnel: w444 -> [w460]
                  tunnel: w443 -> [w458]
                  tunnel: [w457] -> w439
                  tunnel: w438 -> [w459]
                  tunnel: w435 -> [w456]
                  tunnel: w434 -> [w455] mode=indexing
                  tunnel: w432 -> [_]
                  tunnel: w431 -> [w454]
                  tunnel: w430 -> [w453] mode=indexing
                  tunnel: w429 -> [w452]
                  tunnel: [w451] -> w428
                  i -> [w464]
                  stop <- w462 stop-if-true
                  n140 = Increment(x=w464) -> (x+1=w463:i32)
                  n141 = call "motor_move_position.vi"("磁铁最低位置"=w456, "target position"=w455, "device index"=w459) -> ("错误输出"=w451:errorcluster)  [unwired: 6 in, 2 out]
                  n142 = Equal?(x=w465, y=w463) -> (x = y?=w461:bool)
                  n143 = property class="DigNum (strict)"(reference=w460, "Value"=w455) -> ()  [unwired: 1 in, 2 out]
                  n144 = call "REC_wait.vi"("暂停磁铁引用"=w452, "时间单位"=w454, "停止测量引用"=w458, "停留时间"=w453) -> ("停止？"=w457:bool)  [unwired: 7 in]
                  n145 = Or(x=w457, y=w461) -> (x .or. y?=w462:bool)
                }
                n146 = case shown="True" w427 {
                  tunnel: w428 -> [w446 w450]
                  tunnel: [w446 w450] -> _
                  tunnel: w426 -> [_ w447]
                  frame False {
                  }
                  frame True {
                    n147 = Multiply(x=w447, y=u32 1000) -> (x*y=w448:u32)
                    n148 = Wait (ms)(milliseconds to wait=w448) -> ()  [unwired: 1 out]
                  }
                }
                n149 = Select(t=磁铁进程控制变量."返回运动", s=w437, f=磁铁进程控制变量."完成检查") -> (s? t:f=w440:T5)
              }
              frame "返回运动" {
                n150 = Array Size(array=w470) -> (size(s)=w479:i32)
                n151 = Reverse 1D Array(array=w470) -> (reversed array=w480:dbl[])
                n152 = Reverse 1D Array(array=w466) -> (reversed array=w467:dbl[])
                n153 = while {
                  tunnel: [w487] -> w478
                  tunnel: w480 -> [w485] mode=indexing
                  tunnel: w479 -> [w491]
                  tunnel: w477 -> [w490]
                  tunnel: w476 -> [w488]
                  tunnel: w475 -> [w489]
                  tunnel: w472 -> [w486]
                  tunnel: w469 -> [w484]
                  tunnel: w467 -> [w483] mode=indexing
                  tunnel: w468 -> [w482]
                  tunnel: [w481] -> _
                  i -> [w495]
                  stop <- w493 stop-if-true
                  n154 = call "motor_move_position.vi"("磁铁最低位置"=w486, "target position"=w485, "device index"=w490) -> ("错误输出"=w481:errorcluster)  [unwired: 6 in, 2 out]
                  n155 = Increment(x=w495) -> (x+1=w494:i32)
                  n156 = Equal?(x=w491, y=w494) -> (x = y?=w492:bool)
                  n157 = property class="DigNum (strict)"(reference=w489, "Value"=w485) -> ()  [unwired: 1 in, 2 out]
                  n158 = call "REC_wait.vi"("暂停磁铁引用"=w482, "时间单位"=w484, "停止测量引用"=w488, "停留时间"=w483) -> ("停止？"=w487:bool)  [unwired: 7 in]
                  n159 = Or(x=w487, y=w492) -> (x .or. y?=w493:bool)
                }
              }
              frame "完成检查" {
                # "等待10s好判断回归位置"
                n160 = call "motor_move_position.vi"("磁铁最低位置"=w500, "target position"=w499, "device index"=w501) -> ()  [unwired: 6 in, 3 out]
                n161 = property class="DigNum (strict)"(reference=w498, "Value"=w499) -> ()  [unwired: 1 in, 2 out]
                n162 = Increment(x=w508) -> (x+1=w504:i32)
                n163 = Wait (ms)(milliseconds to wait=u32 10000) -> ()  [unwired: 1 out]
                n164 = Equal?(x=w503, y=w504) -> (x = y?=w502:bool)
                n165 = call "warning tone.vi"("Ring?"=TRUE) -> ()  [unwired: 11 in]
              }
            }
            n166 = Or(x=w368, y=w373) -> (x .or. y?=w376:bool)
          }
        }
        frame "user-defined" {
          n167 = while {
            tunnel: w512 -> [w515]
            tunnel: [w513] -> w511
            stop <- w513 stop-if-true
            n168 = property class="Bool (strict)"(reference=w515) -> ("Value"=w513:bool)  [unwired: 1 in, 2 out]
            n169 = Wait (ms)(milliseconds to wait=u32 1000 ("millisecond timer value")) -> ()  [unwired: 1 out]
          }
        }
      }
    }
    frame True {
    }
  }
  "完成测量" <- w3
